vi "AlliGator Remove Selected Phasor Plots.vi"(8 "error in (no error)":errorcluster, 9 "Phasor Reference 1 Refnum":refnum<vi>, 10 "Selected Plot Info":T1, 11 "AlliGator IV DVR in":refnum<data-value>) -> (0 "error out":errorcluster, 2 "Message":string, 3 "AlliGator IV DVR out":refnum<data-value>)   [LabVIEW 2021, in "AlliGator Phasor Graph.lvlib"]
doc: "Removes selected Phasor Plots from Phasor Graph.\n\nNote that other actions need to be performed to remove the associated data and metadata."
uses:
  AlliGator Phasor Graph.lvlib
  Graphs/XY Graph/XY Graph Selected Plot Info.ctl
  Graphs/XY Graph/XY Graph Refnum.ctl
  <vilib>/Utility/miscctls.llb/LVPoint32TypeDef.ctl
  AlliGator Internal Variables v2.ctl
  <vilib>/vision/Image Controls.llb/IMAQ Image.ctl
  AlliGator Gate Image Set.ctl
  AlliGator FLI Dataset Type.ctl
  AlliGator Data Series Type.ctl
  AlliGator Dataset Channel.ctl
  AlliGator Gate Arithmetic.ctl
  AlliGator Displayed Image.ctl
  Image/Named ROI Description.ctl
  AlliGator Decay Metadata v3.ctl
  AlliGator Decay Background Subtraction Info.ctl
  AlliGator Baseline Subtraction Method.ctl
  Graphs/XY Graph/XY Graph Plot Shift Parameters.ctl
  Graphs/XY Graph/XY Graph Plot Shift Method.ctl
  AlliGator Decay Extrapolation Parameters.ctl
  Phasor/Calibration Phasor (m, phi).ctl
  Phasor/Phasor Reference Series.ctl
  Phasor/Phasor Calibration Map v2.ctl
  Phasor/Phasor (g, s).ctl
  AlliGator Raw Phasor Plot Data v4.ctl
  Phasor/Phasor Standard Deviation Options.ctl
  AlliGator Phasor Multi-Harmonic Data.ctl
  Phasor/Phasor Harmonic Data.ctl
  AlliGator Decay Fit Options & Parameters v2.ctl
  Fits/IRF(X)PSED/Decay Fit Options v2.ctl
  Fits/Decay Convolution/Decay Model.ctl
  Fits/Residual Type.ctl
  Fits/IRF(X)PSED/Fit Weights Type.ctl
  Fits/Non-linear Fitting Method v2.ctl
  Fits/Fit Calculation Method.ctl
  Fits/Non-linear Fitting Algorithm.ctl
  AlliGator Decay Fit Parameter Constraints 2.ctl
  Fits/IRF(X)PSED/Decay Fit Parameters In List.ctl
  Fits/IRF(X)PSED/MLE Baseline Offset Type.ctl
  AlliGator Decay Preprocessing Parameters.ctl
  Fits/IRF(X)PSED/Decay Fit Parameters & Derived Quantities List.ctl
  026df5fa-8ed4-4270-81a2-1ef72d82da0f.vi
  <userlib>/_OpenG.lib/array/array.llb/Filter 1D Array with Scalar (I32)__ogtk.vi
  <vilib>/Comparison/Less/Less Functor/Less Functor.lvclass
  AlliGator Phasor Calibration.lvlib
  Graphs/XY Graph/XY Graph Add-Ons.lvlib
  <userlib>/_OpenG.lib/array/array.llb/openg_array.lvlib
  Strings/Strings.lvlib
  AlliGator Source Image.lvlib
  Phasor/Phasor.lvlib
  Image/Image.lvlib
  AlliGator Decay Preprocessing.lvlib
  AlliGator Files.lvlib
  AlliGator Phasor Plot.lvlib
  Fits/Fits.lvlib
  AlliGator Decay Fit.lvlib
  AlliGator Decay Fit Parameter Map.lvlib
  AlliGator Settings.lvlib
  AlliGator Dual-Channel Datasets.lvlib
  AlliGator Internal Variables.lvlib
panel:
  # "see the AlliGator License on the block diagram (Ctrl+E or Window:Show Block Diagram)"
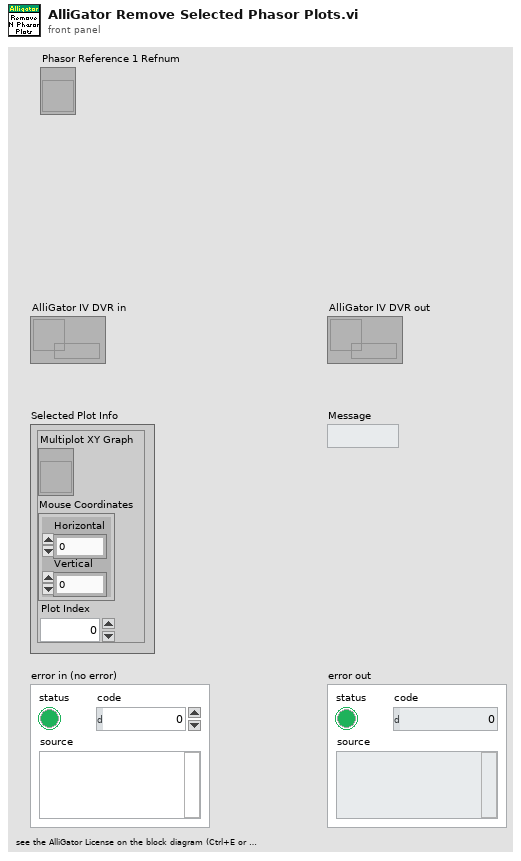
[diagram p1: front panel]
types:
  T1 = typedef "XY Graph Add-Ons.lvlib/XY Graph Selected Plot Info.ctl" = cluster{"Multiplot XY Graph":T2, "Mouse Coordinates":T3, "Plot Index":i32}
  T2 = typedef "XY Graph Add-Ons.lvlib/XY Graph Refnum.ctl" = refnum<vi>
  T3 = typedef "LVPoint32TypeDef.ctl" = cluster{"Horizontal":i32, "Vertical":i32}
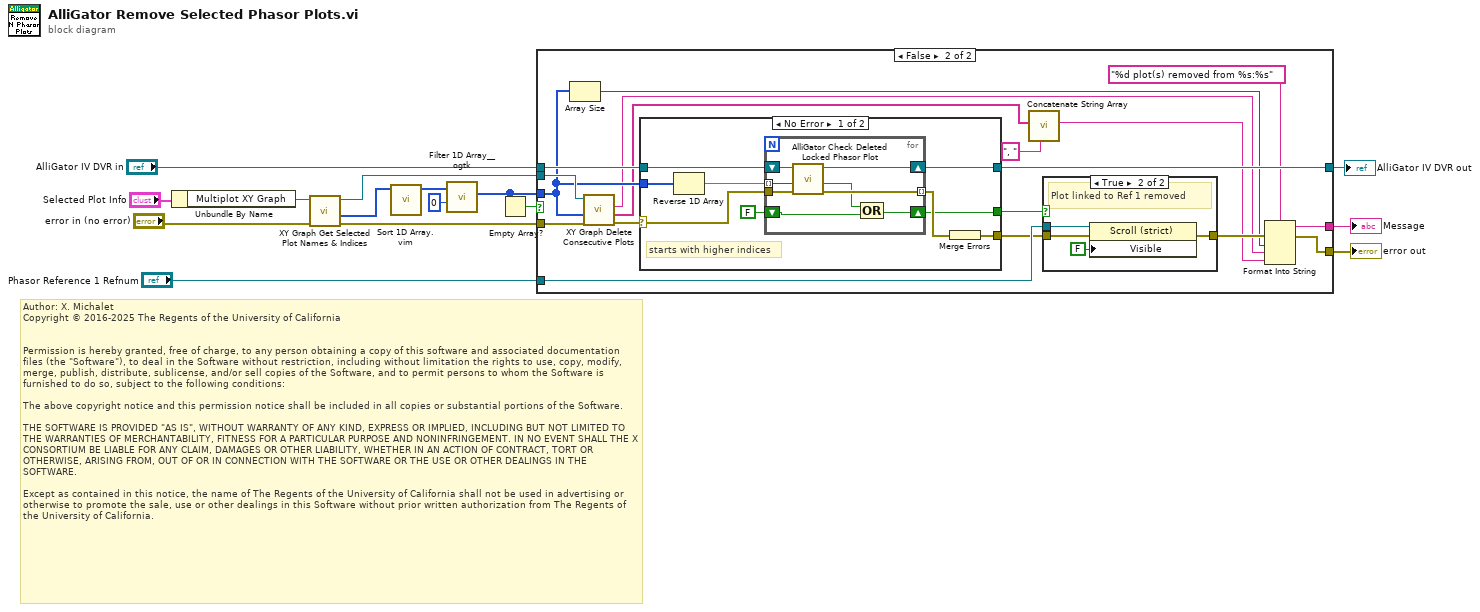
[diagram p0: block diagram]
diagram:
  # "Author: X. Michalet\nCopyright © 2016-2025 The Regents of the University of California\n \n\nPermission is hereby granted, free of charge, to any person obtaining a copy of this software and associated documentation files (the \"Software\"), to deal in the Software without restriction, including without limitation the rights to use, copy, modify, merge, publish, distribute, sublicense, and/or sell copies of the Software, and to permit persons to whom the Software is furnished to do so, subject to the following conditions:\n\nThe above copyright notice and this permission notice shall be included in all copies or substantial portions of the Software.\n\nTHE SOFTWARE IS PROVIDED \"AS IS\", WITHOUT WARRANTY OF ANY KIND, EXPRESS OR IMPLIED, INCLUDING BUT NOT LIMITED TO THE WARRANTIES OF MERCHANTABILITY, FITNESS FOR A PARTICULAR PURPOSE AND NONINFRINGEMENT. IN NO EVENT SHALL THE X CONSORTIUM BE LIABLE FOR ANY CLAIM, DAMAGES OR OTHER LIABILITY, WHETHER IN AN ACTION OF CONTRACT, TORT OR OTHERWISE, ARISING FROM, OUT OF OR IN CONNECTION WITH THE SOFTWARE OR THE USE OR OTHER DEALINGS IN THE SOFTWARE.\n\nExcept as contained in this notice, the name of The Regents of the University of California shall not be used in advertising or otherwise to promote the sale, use or other dealings in this Software without prior written authorization from The Regents of the University of California."
  n1 = Unbundle By Name("Selected Plot Info") -> ("Multiplot XY Graph"=w10:T2)
  n2 = call "XY Graph Get Selected Plot Names & Indices.vi"("error in (no error)"="error in (no error)", "XYGraph in"=w10) -> ("error out"=w8:errorcluster, "Selected Plots"=w5:i32[], "XYGraph out"=w6:T2)  [unwired: 5 in, 2 out]
  n3 = call "Sort 1D Array.vim"("unsorted array"=w5) -> ("sorted array"=w4:i32[])  [unwired: 10 in]
  n4 = call-poly <userlib>:"Filter 1D Array__ogtk.vi"("items to filter"=0, "array"=w4) -> ("filtered array"=w2:i32[])  [unwired: 4 in, 1 out]
  n5 = Empty Array?(array=w2) -> (empty?=w7:bool)
  n6 = case shown="False" w7 {
    tunnel: "AlliGator IV DVR in" -> [w17 w35]
    tunnel: [w17 w34] -> w13
    tunnel: w8 -> [w16 w30]
    tunnel: [w16 w26] -> w15
    tunnel: "Phasor Reference 1 Refnum" -> [_ w33]
    tunnel: w6 -> [_ w28]
    tunnel: w2 -> [_ w23]
    tunnel: [_ w24] -> w1
    frame True {
    }
    frame False {
      n7 = Array Size(array=w23) -> (size(s)=w22:i32)
      n8 = call "XY Graph Delete Consecutive Plots.vi"("Error In"=w30, "Plot Indices"=w23, "XYGraph Ref"=w28) -> ("Error Out"=w29:errorcluster, "Plot Names"=w20:string[], "Graph Caption (or Label)"=w21:string)  [unwired: 5 in, 1 out]
      n9 = case shown="No Error" w29 {
        selector: w29 -> [w40 w53]
        tunnel: w35 -> [w42 w54]
        tunnel: [w41 w54] -> w34
        tunnel: [w38 w53] -> w32
        tunnel: [w43 _] -> w31
        tunnel: w23 -> [w37 _]
        frame No Error {
          # "starts with higher indices"
          n10 = Reverse 1D Array(array=w37) -> (reversed array=w36:i32[])
          n11 = for {
            tunnel: [w52] -> w44 mode=indexing
            shift-right: [w49] -> w41
            shift-left: w42 -> [w50]
            tunnel: w40 -> [w48]
            shift-right: [w47] -> w43
            shift-left: FALSE -> [w46]
            tunnel: w36 -> [w45] mode=indexing
            n12 = call "AlliGator Check Deleted Locked Phasor Plot.vi"("Error In"=w48, "Deleted Plot Index"=w45, "AlliGator Internal Variables DVR"=w50) -> ("Error Out"=w52:errorcluster, "Hide Reference 1 Control"=w51:bool, "AlliGator Internal Variables DVR"=w49:refnum<data-value>)  [unwired: 6 in]
            n13 = Compound Arithmetic op=OR(w51, w46) -> (w47:bool)
          }
          n14 = Merge Errors(w44) -> (w38:errorcluster)
        }
        frame Error {
        }
      }
      n15 = call "Concatenate String Array.vi"("Separator (TAB)"=", ", "String Array"=w20) -> ("Formatted String"=w18:string)  [unwired: 9 in]
      n16 = case shown="True" w31 {
        tunnel: w33 -> [_ w59]
        tunnel: w32 -> [w55 w58]
        tunnel: [w55 w57] -> w27
        frame False {
        }
        frame True {
          # "Plot linked to Ref 1 removed"
          n17 = property class="Scroll (strict)"(reference=w59, error in=w58, "Visible"=FALSE) -> (error out=w57:errorcluster)  [unwired: 1 out]
        }
      }
      n18 = Format Into String(format string="%d plot(s) removed from %s:%s", error in=w27, w22, w21, w18) -> (resulting string=w24:string, error out=w26:errorcluster)  [unwired: 1 in]
    }
  }
  "Message" <- w1
  "error out" <- w15
  "AlliGator IV DVR out" <- w13
